vi "GasSensor_Final.vi"() -> ()   [LabVIEW 2022 SP3]
uses:
  <vilib>/DAQmx/read.llb/DAQmx Read (Analog DBL 1Chan 1Samp).vi
  <vilib>/DAQmx/create/channels.llb/DAQmx Create Channel (AI-Voltage-Basic).vi
  <vilib>/DAQmx/miscellaneous.llb/DAQmx Fill In Error Info.vi
panel:
  out "String":string
  in  "stop":bool
  out "Meter":dbl(knob) scale=0.0..3.0
  in  "DAQmx Physical Channel":tag
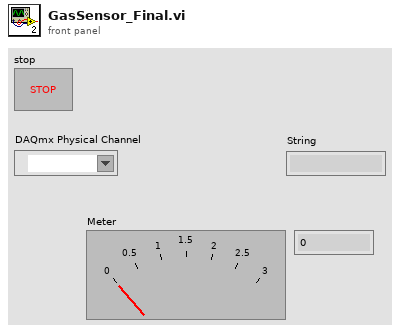
[diagram p1: front panel]
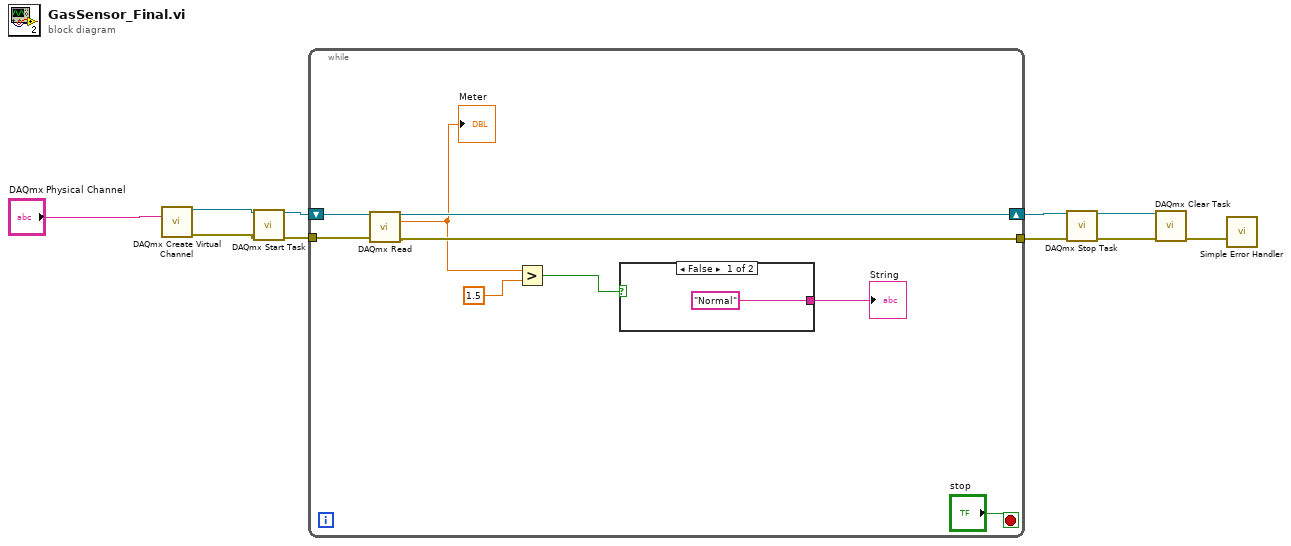
[diagram p0: block diagram]
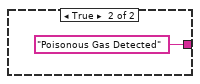
[diagram p2: hidden frame]
diagram:
  n1 = call-poly <vilib>:"DAQmx Create Virtual Channel.vi"("physical channels"="DAQmx Physical Channel") -> ("task out"=w5:refnum<k21>, "error out"=w4:errorcluster)  [unwired: 13 in]
  n2 = call <vilib>:"DAQmx Start Task.vi"("task/channels in"=w5, "error in"=w4) -> ("task out"=w3:refnum<k21>, "error out"=w2:errorcluster)  [unwired: 12 in]
  n3 = while {
    tunnel: w2 -> [w17]
    shift-right: [w19] -> w9
    shift-left: w3 -> [w18]
    tunnel: [w15] -> w1
    stop <- "stop" stop-if-true
    n4 = call-poly <vilib>:"DAQmx Read.vi"("task/channels in"=w18, "error in"=w17) -> ("task out"=w19:refnum<k21>, "data"=w14:dbl, "error out"=w15:errorcluster)  [unwired: 11 in]
    "Meter" <- w14
    n5 = Greater?(x=w14, y=1.5) -> (0:w12:bool)
    n6 = case shown="False" w12 {
      tunnel: ["Normal" "Poisonous Gas Detected"] -> w11
      frame False {
      }
      frame True {
      }
    }
    "String" <- w11
  }
  n7 = call <vilib>:"DAQmx Stop Task.vi"("task/channels in"=w9, "error in"=w1) -> ("task out"=w8:refnum<k21>, "error out"=w7:errorcluster)  [unwired: 12 in]
  n8 = call <vilib>:"DAQmx Clear Task.vi"("task in"=w8, "error in"=w7) -> ("error out"=w6:errorcluster)  [unwired: 13 in]
  n9 = call <vilib>:"Simple Error Handler.vi"("error in (no error)"=w6) -> ()  [unwired: 4 in, 5 out]
